vi "Auto Collimation Process.vi"(8 "error in (no error)":errorcluster, 11 "Fiber Auto Collimation state data in":refnum<class "Fiber Auto Collimation state data.lvclass">) -> (0 "error out":errorcluster, 3 "Fiber Auto Collimation state data out":refnum<class "Fiber Auto Collimation state data.lvclass">)   [LabVIEW 2018]
uses:
  State data/Fiber Auto Collimation state data.lvclass
  <userlib>/nLight Tidbits/Logging/Controls/Logging type choice.ctl
  State data/Fiber Auto Collimation state data.lvclass/Fiber Auto Collimation state data.ctl
  State data/Add Changed data.vi
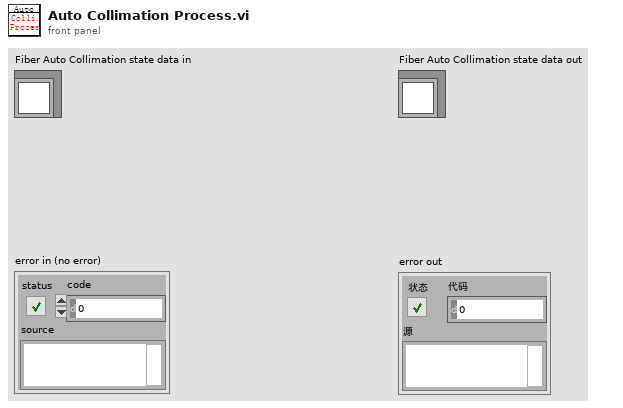
[diagram p1: front panel]
types:
  T1 = typedef "Logging type choice.ctl" = enum16{"No log type selected", "Testing start/stop", "Test progress", "Station startup/shutdown", "Station config change", "Recipe load/change", "Inventory transaction", "Instrument", "Debug"}
  T2 = typedef "Fiber Auto Collimation state data.lvclass/BV Data.ctl" = cluster{"Centroid X[um]":sgl, "Centroid Y[um]":sgl, "PeakResp.[%]":dbl, "Knife Edge X[mm]":sgl, "Knife Edge Y[mm]":sgl, "Circularity":sgl, "Collimation Result":bool}
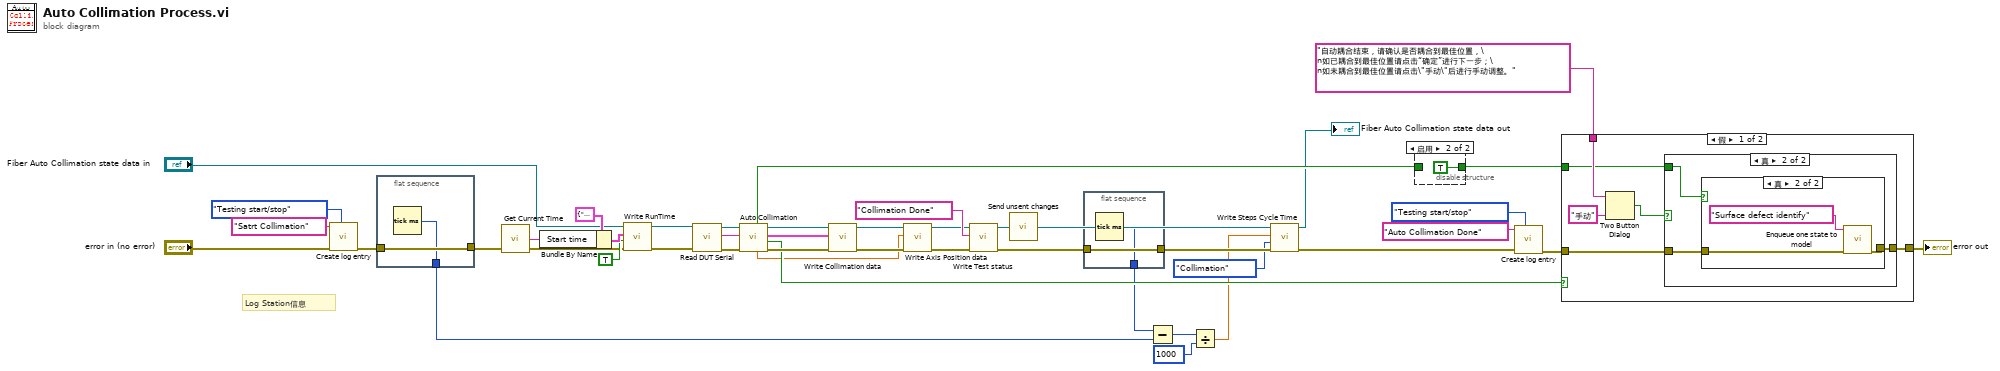
[diagram p0: block diagram]
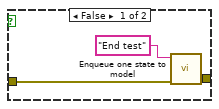
[diagram p3: hidden frame]
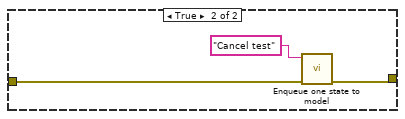
[diagram p4: hidden frame]
diagram:
  # "Log Station信息"
  n1 = call <userlib>:"Create log entry.vi"("Logging type choice"=Logging_type_choice."Testing start/stop", "error in (no error)"="error in (no error)", "Brief log entry"="Satrt Collimation") -> ("error out"=w19:errorcluster)  [unwired: 8 in]
  n2 = flat-sequence {
    tunnel: w19 -> [w46]
    tunnel: [w46] -> w18
    tunnel: [w45] -> w15
    frame #0 {
      n3 = Tick Count (ms)() -> (millisecond timer value=w45:u32)
    }
  }
  n4 = call "Get Current Time.vi"() -> ("日期/时间字符串"=w31:string)  [unwired: 1 in]
  n5 = Bundle By Name(cluster=cluster{"Start time":string, "End time":string} {"Start time"="", "End time"=""} ("Run Time"), "Start time"=w31) -> (w32:cluster{"Start time":string, "End time":string})
  n6 = call "Write RunTime.vi"("error in (no error)"=w18, "Start time"=TRUE, "Run Time"=w32, "Fiber Auto Collimation state data in"="Fiber Auto Collimation state data in") -> ("error out"=w1:errorcluster, "Fiber Auto Collimation state data out"=w20:refnum<class "Fiber Auto Collimation state data.lvclass">)  [unwired: 6 in]
  n7 = call "Read DUT Serial.vi"("error in (no error)"=w1, "Fiber Auto Collimation state data in"=w20) -> ("error out"=w40:errorcluster, "DUT Serial"=w25:string, "Fiber Auto Collimation state data out"=w30:refnum<class "Fiber Auto Collimation state data.lvclass">)  [unwired: 7 in]
  n8 = call "Auto Collimation.vi"("error in (no error)"=w40, "SN"=w25, "Fiber Auto Collimation state data in"=w30) -> ("error out"=w36:errorcluster, "Cancel Test"=w26:bool, "BV Data"=w41:T2, "Fiber Auto Collimation state data out"=w27:refnum<class "Fiber Auto Collimation state data.lvclass">, "Stop Position"=w2:dbl[unit], "Collimation result"=w28:bool)  [unwired: 3 in]
  n9 = call "Write Collimation data.vi"("error in (no error)"=w36, "BV Data"=w41, "Fiber Auto Collimation state data in"=w27) -> ("error out"=w6:errorcluster, "Fiber Auto Collimation state data out"=w4:refnum<class "Fiber Auto Collimation state data.lvclass">)  [unwired: 7 in]
  n10 = call "Write Axis Position data.vi"("error in (no error)"=w6, "Current Position"=w2, "Fiber Auto Collimation state data in"=w4) -> ("error out"=w5:errorcluster, "Fiber Auto Collimation state data out"=w3:refnum<class "Fiber Auto Collimation state data.lvclass">)  [unwired: 7 in]
  n11 = call "Write Test status.vi"("error in (no error)"=w5, "Test status"="Collimation Done", "Fiber Auto Collimation state data in"=w3) -> ("error out"=w17:errorcluster, "Fiber Auto Collimation state data out"=w44:refnum<class "Fiber Auto Collimation state data.lvclass">)  [unwired: 7 in]
  n12 = call "Send unsent changes.vi"("Fiber Auto Collimation state data in"=w44) -> ("Fiber Auto Collimation state data out"=w10:refnum<class "Fiber Auto Collimation state data.lvclass">)  [unwired: 1 in]
  n13 = flat-sequence {
    tunnel: w17 -> [w48]
    tunnel: [w48] -> w12
    tunnel: [w47] -> w16
    frame #0 {
      n14 = Tick Count (ms)() -> (millisecond timer value=w47:u32)
    }
  }
  n15 = Subtract(x=w16, y=w15) -> (x-y=w14:u32)
  n16 = Divide(x=w14, y=u32 1000) -> (x/y=w11:dbl)
  n17 = call "Write Steps Cycle Time.vi"("error in (no error)"=w12, "Steps Action"=enum16{"Collimation", "Defect detection"}."Collimation", "Cycle Time"=w11, "Fiber Auto Collimation state data in"=w10) -> ("error out"=w7:errorcluster, "Fiber Auto Collimation state data out"=→"Fiber Auto Collimation state data out":refnum<class "Fiber Auto Collimation state data.lvclass">)  [unwired: 6 in]
  n18 = disable-structure shown="启用" {
    disable-tunnel: w28 -> [w49 _]
    disable-tunnel: [w49 TRUE] -> w42
    frame Disabled {
    }
    frame Enabled {
    }
  }
  n19 = call <userlib>:"Create log entry.vi"("Logging type choice"=Logging_type_choice."Testing start/stop", "error in (no error)"=w7, "Brief log entry"="Auto Collimation Done") -> ("error out"=w34:errorcluster)  [unwired: 8 in]
  n20 = case shown="假" w26 {
    tunnel: [w56 w67] -> w23
    tunnel: w42 -> [w52 _]
    tunnel: w34 -> [w55 w68]
    tunnel: "自动耦合结束，请确认是否耦合到最佳位置，\n如已耦合到最佳位置请点击“确定”进行下一步；\n如未耦合到最佳位置请点击\"手动\"后进行手动调整。" ("message") -> [w54 _]
    frame False {
      n21 = Two Button Dialog(message=w54, 1:"手动" ("F按钮名称（“取消”）")) -> (T button?=w51:bool)  [unwired: 1 in]
      n22 = case shown="真" w51 {
        tunnel: [w57 w60] -> w56
        tunnel: w55 -> [w57 w59]
        tunnel: w52 -> [_ w58]
        frame False {
        }
        frame True {
          n23 = case shown="真" w58 {
            tunnel: [w61 w65] -> w60
            tunnel: w59 -> [w62 w64]
            frame False {
              n24 = call "Enqueue one state to model.vi"("error in (no error)"=w62, "Enqueued state"="End test") -> ("error out"=w61:errorcluster)  [unwired: 9 in]
            }
            frame True {
              n25 = call "Enqueue one state to model.vi"("error in (no error)"=w64, "Enqueued state"="Surface defect identify") -> ("error out"=w65:errorcluster)  [unwired: 9 in]
            }
          }
        }
      }
    }
    frame True {
      n26 = call "Enqueue one state to model.vi"("error in (no error)"=w68, "Enqueued state"="Cancel test") -> ("error out"=w67:errorcluster)  [unwired: 9 in]
    }
  }
  "error out" <- w23
